vi "accept_connection.vi"(4 "WebSocket Logger":refnum<class "WebSocket Logger.lvclass">, 6 "Sec-WebSocket-Protocol":string[](array[string]), 8 "error in (no error)":errorcluster, 9 "remote address":string, 10 "remote port":u16, 11 "WebSocket Connection Handler in":refnum<class "WebSocket Connection Handler.lvclass">) -> (0 "error out":errorcluster, 1 "accept connection?":bool, 2 "Sec-WebSocket-Protocol accepted":string, 3 "WebSocket Connection Handler out":refnum<class "WebSocket Connection Handler.lvclass">)   [LabVIEW 2019, in "WebSocket Server Toolkit.lvlib" / "WebSocket Connection Handler.lvclass"]
doc: "<b>Description</b> Override this VI to selectively accept connections.\n\n<b>Inputs</b>\n<b>Sec</b>: -WebSocket-Protocol\nRequested protocols.\n<b>remote address</b>: Peer address\n<b>remote port</b>: The port the client is connecting from.\n\n<b>Outputs</b>\n<b>Sec</b>: -WebSocket-Protocol accepted\nAccepted protocol."
uses:
  WebSocket Connection Handler.lvclass
  WebSocket Logger/WebSocket Logger.lvclass
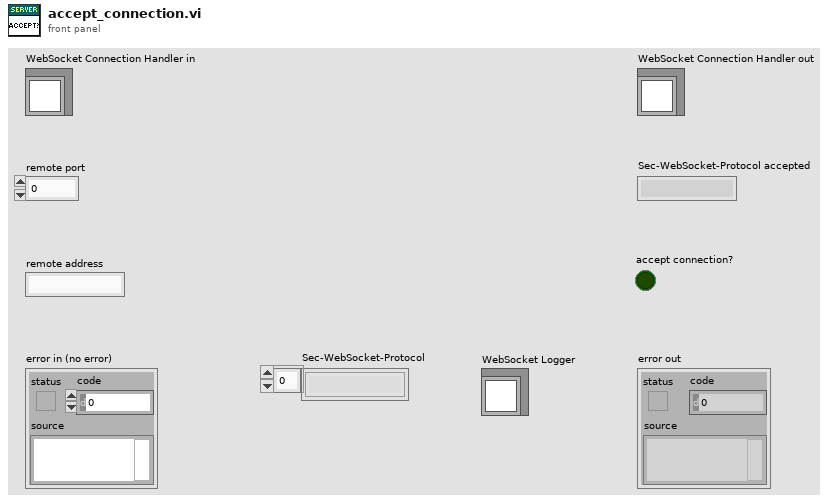
[diagram p1: front panel]
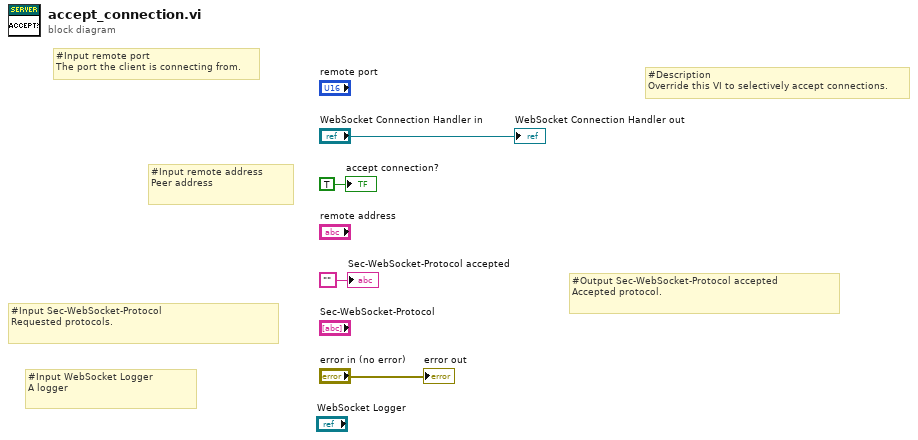
[diagram p0: block diagram]
diagram:
  # "#Input WebSocket Logger\nA logger"
  # "#Output Sec-WebSocket-Protocol accepted\nAccepted protocol."
  # "#Input Sec-WebSocket-Protocol\nRequested protocols."
  # "#Input remote address\nPeer address"
  # "#Input remote port\nThe port the client is connecting from."
  # "#Description\nOverride this VI to selectively accept connections."
  "error out" <- "error in (no error)"
  "WebSocket Connection Handler out" <- "WebSocket Connection Handler in"
  "Sec-WebSocket-Protocol accepted" <- ""
  "accept connection?" <- TRUE ("accept connection?")
